vi "LinearSystemLoop_DiffDrv_Execute.vi"(5 "Linear System":T2, 6 "dT_Seconds":dbl=0.02 format="%#_13g", 7 "LinearSystemLoop_DiffDrv_Control_Params":T1={"Left Vel Model Std Dev m/s"=0.0, "Left Vel Meas Std Dev m/s"=0.0, "Left Vel Ctrl Tol m/s"=0.0, "Max Control Effort"=12.0, "Right Vel Ctrl Tol m/s"=0.0, "Right Vel Meas Std Dev m/s"=0.0, "Right Vel Model Std Dev m/s"=0.0}, 8 "Right Vel PV m/s":dbl, 9 "Left Vel PV m/s":dbl, 10 "Right Vel SP m/s":dbl, 11 "Left Vel SP m/s":dbl) -> (0 "Error":bool, 1 "Filtered Measurements":dbl[](array[numeric]), 2 "Right Motor Dmd":dbl, 3 "Left Motor Dmd":dbl, 4 "out Linear System Loop":T4)   [LabVIEW 2019, in "Trajectory_Library.lvlib"]
doc: "The linear system is define as:\n - states\n - left velocity (m/s)\n - right velocity (m/s)\n - inputs\n - left voltage (volts)\n - right voltage(volts)\n - outputs\n - left velocity (m/s)\n - right velocity (m/s)"
uses:
  Trajectory_Library.lvlib
  TypeDef/LINEAR_SYSTEM_LOOP.ctl
  TypeDef/LINEAR_QUADRATIC_REGULATOR.ctl
  <vilib>/Analysis/Matrix/Datatypes/RealMatrix.ctl
  TypeDef/LINEAR_PLANT_INV_FF.ctl
  TypeDef/KALMAN_FILTER.ctl
  TypeDef/LINEAR_SYSTEM.ctl
  TypeDef/LINEAR_SYSTEM_LOOP_DIFF_DRV_CTRL_PARAMS.CTL
  MatBuilder_Create.vi
  <vilib>/Analysis/Matrix/Numeric/Conversions/Matrix To Array - RM.vi
  <vilib>/Analysis/Matrix/NI_Matrix.lvlib
panel:
  # "<States,States>"
  # "<States,Inputs>"
  # "<Outputs,States>"
  # "<Outputs,Inputs>"
  # "<States,1>"
  # "<FUTURE --- CLAMP TYPE -- For now\nuse Normalize>"
  # "Steady State Gain  \n<States,Outputs>"
  # "State Estimate <Statess,1>"
  # "<States,States>"
  # "<States,Inputs>"
  # "<Outputs,States>"
  # "<Outputs,Inputs>"
  # "<States,1>"
  # "<Inputs,1>"
  # "<States,Inputs>"
  # "<States,States>"
  # "Ref State <States,1>"
  # "Comp and capped \noutput <Inputs,1>"
  # "Controller gain\n<Inputs,States>"
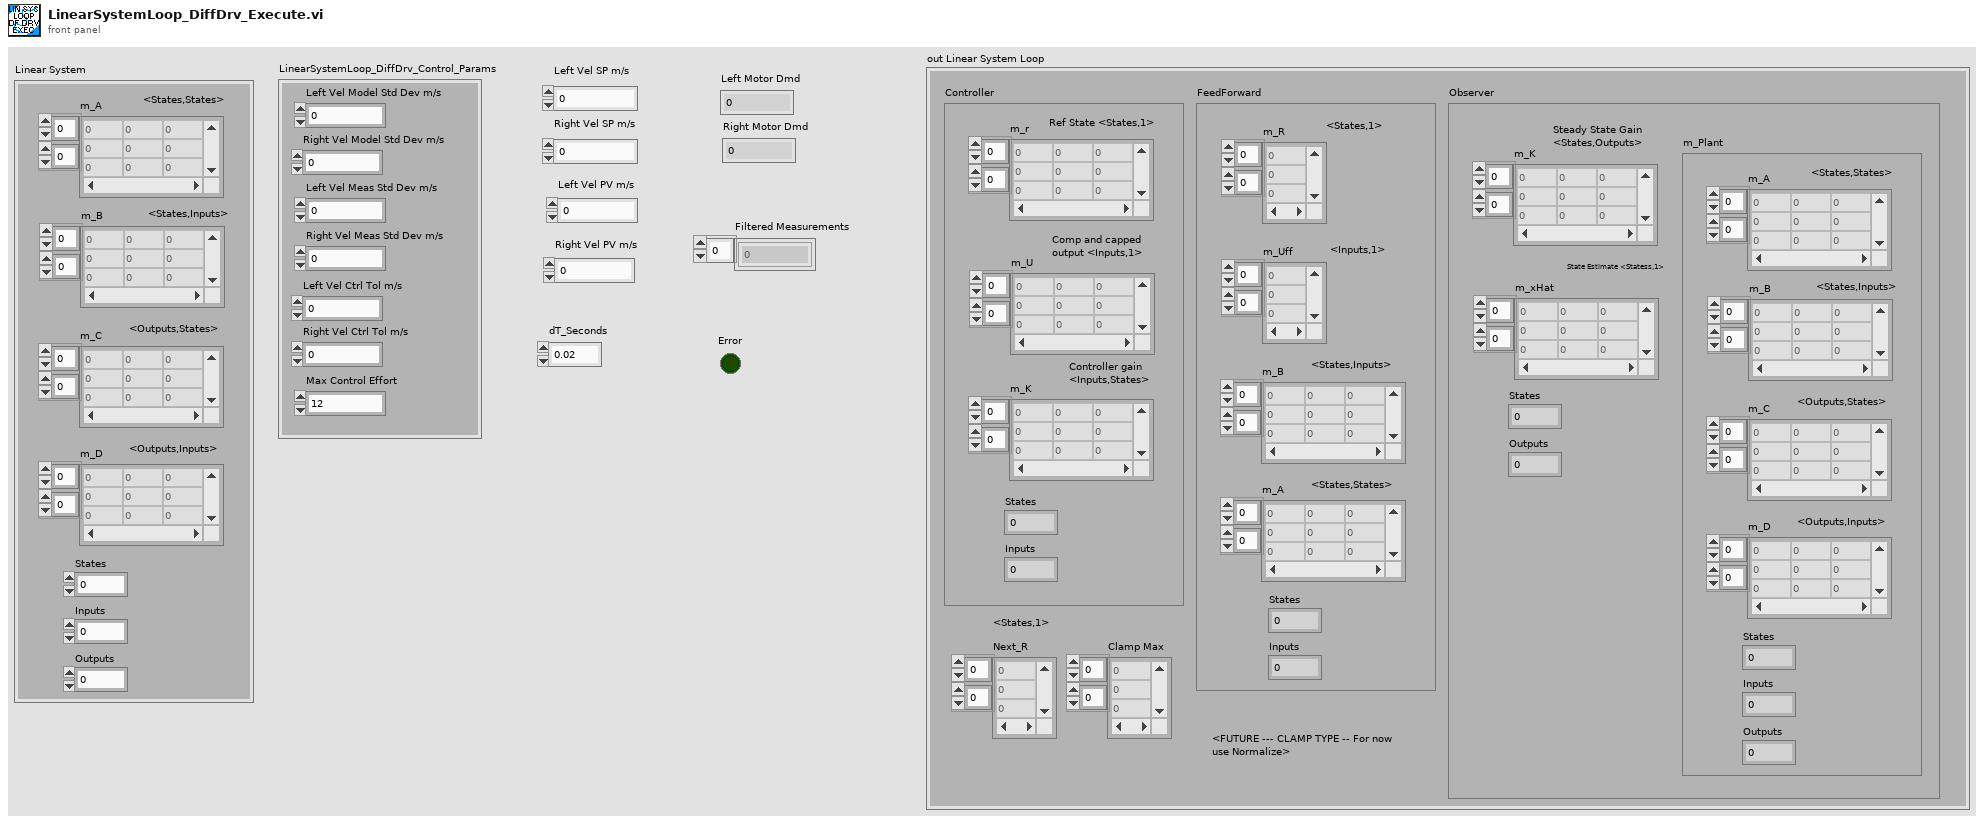
[diagram p1: front panel]
types:
  T1 = typedef "Trajectory_Library.lvlib/LINEAR_SYSTEM_LOOP_DIFF_DRV_CTRL_PARAMS.CTL" = cluster{"Left Vel Model Std Dev m/s":dbl, "Left Vel Meas Std Dev m/s":dbl, "Left Vel Ctrl Tol m/s":dbl, "Max Control Effort":dbl, "Right Vel Ctrl Tol m/s":dbl, "Right Vel Meas Std Dev m/s":dbl, "Right Vel Model Std Dev m/s":dbl}
  T2 = typedef "Trajectory_Library.lvlib/LINEAR_SYSTEM.ctl" = cluster{"m_A":T3, "m_B":T3, "m_C":T3, "m_D":T3, "States":i32, "Inputs":i32, "Outputs":i32}
  T3 = typedef "NI_Matrix.lvlib/RealMatrix.ctl" = dbl[][]
  T4 = typedef "Trajectory_Library.lvlib/LINEAR_SYSTEM_LOOP.ctl" = cluster{"Controller":T5, "FeedForward":T6, "Observer":T7, "Next_R":T3, "Clamp Max":T3}
  T5 = typedef "Trajectory_Library.lvlib/LINEAR_QUADRATIC_REGULATOR.ctl" = cluster{"m_r":T3, "m_U":T3, "m_K":T3, "States":i32, "Inputs":i32}
  T6 = typedef "Trajectory_Library.lvlib/LINEAR_PLANT_INV_FF.ctl" = cluster{"m_R":T3, "m_Uff":T3, "m_B":T3, "m_A":T3, "States":i32, "Inputs":i32}
  T7 = typedef "Trajectory_Library.lvlib/KALMAN_FILTER.ctl" = cluster{"m_K":T3, "m_xHat":T3, "States":i32, "Outputs":i32, "m_Plant":T2}
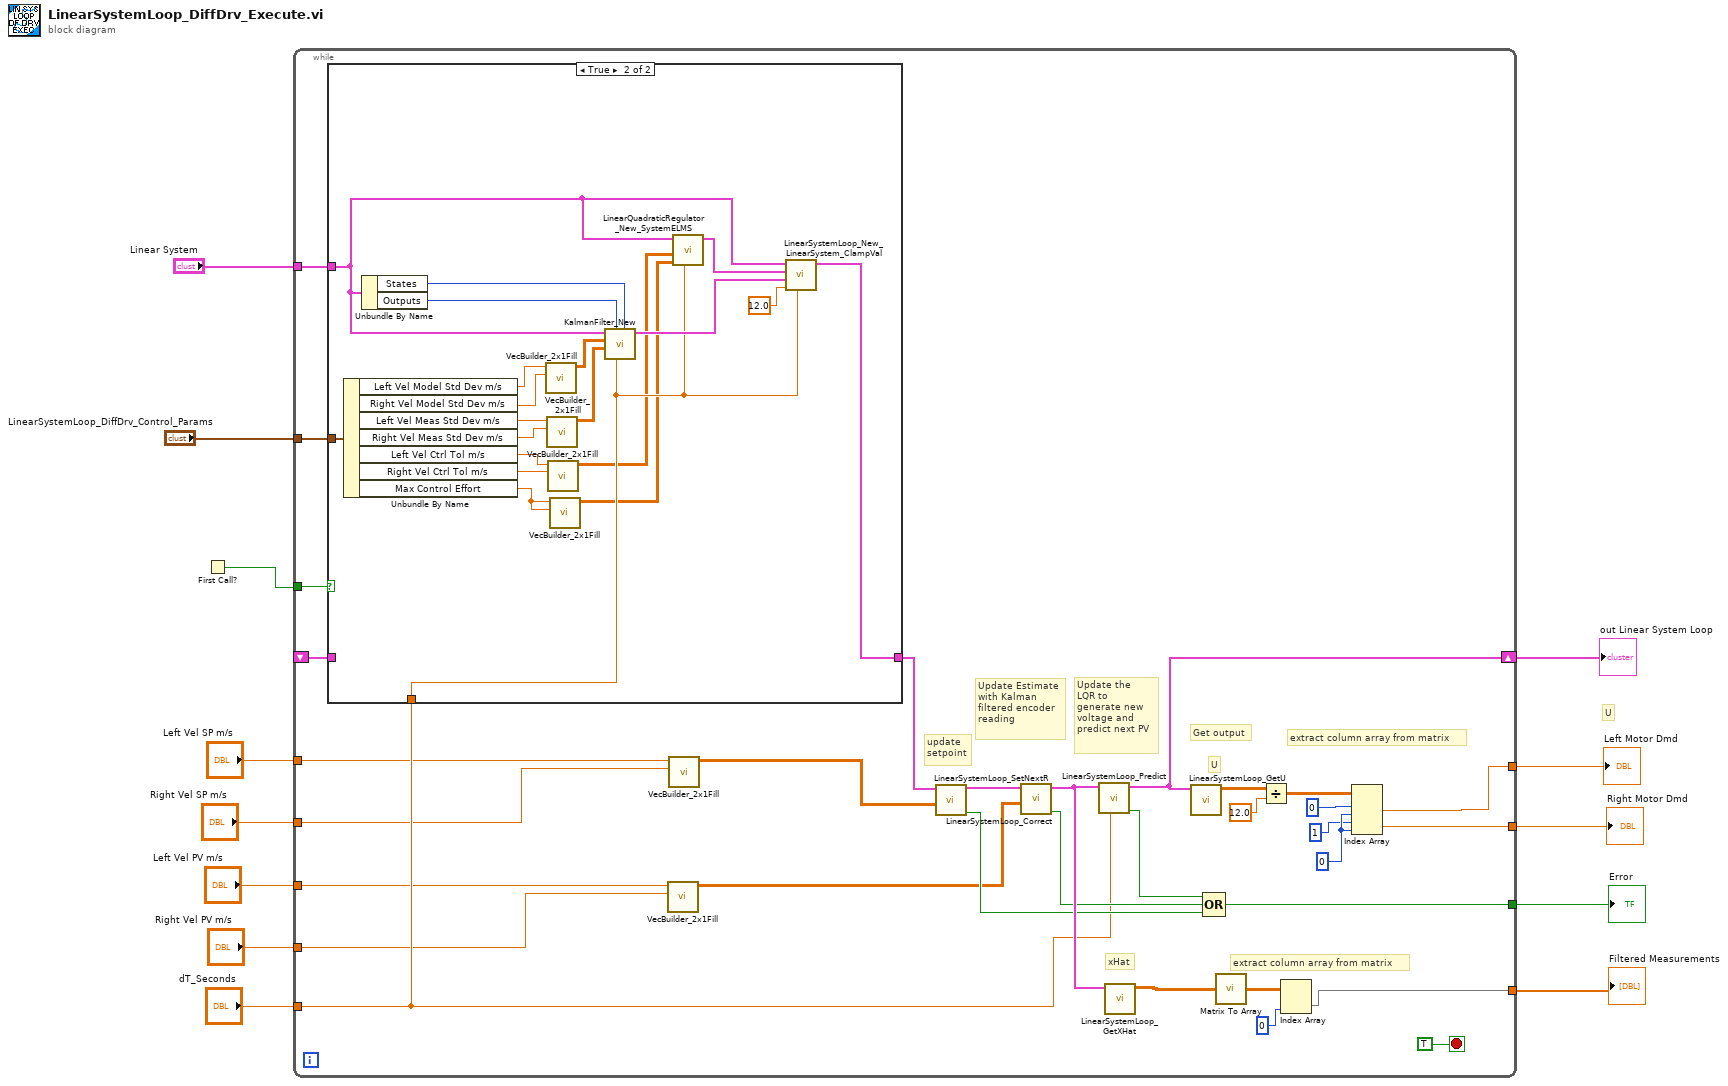
[diagram p0: block diagram]
diagram:
  # "U"
  n1 = First Call?() -> (First Call?: T/F=w9:bool)
  n2 = while {
    tunnel: [w40] -> w12
    tunnel: [w15] -> w7
    tunnel: "Left Vel SP m/s" -> [w24]
    tunnel: "Left Vel PV m/s" -> [w23]
    shift-right: [w44] -> w13
    shift-left: _ -> [w28]
    tunnel: w9 -> [w37]
    tunnel: [w34] -> w8
    tunnel: "dT_Seconds" -> [w29]
    tunnel: "Linear System" -> [w30]
    tunnel: "LinearSystemLoop_DiffDrv_Control_Params" -> [w26]
    tunnel: "Right Vel SP m/s" -> [w25]
    tunnel: "Right Vel PV m/s" -> [w22]
    tunnel: [w14] -> w1
    stop <- TRUE stop-if-true
    w18 = 0 ("index (col)")
    # "extract column array from matrix"
    # "extract column array from matrix"
    # "xHat"
    # "U"
    # "Get output"
    # "Update the \nLQR to \ngenerate new \nvoltage and \npredict next PV"
    # "update \nsetpoint"
    # "Update Estimate\nwith Kalman \nfiltered encoder \nreading"
    n3 = case shown="True" w37 {
      tunnel: [w46 w62] -> w27
      tunnel: w28 -> [w46 _]
      tunnel: w30 -> [_ w65]
      tunnel: w29 -> [_ w61]
      tunnel: w26 -> [_ w59]
      frame False {
      }
      frame True {
        n4 = Unbundle By Name(w59) -> ("Left Vel Model Std Dev m/s"=w57:dbl, "Right Vel Model Std Dev m/s"=w56:dbl, "Left Vel Meas Std Dev m/s"=w55:dbl, "Right Vel Meas Std Dev m/s"=w52:dbl, "Left Vel Ctrl Tol m/s"=w51:dbl, "Right Vel Ctrl Tol m/s"=w50:dbl, "Max Control Effort"=w49:dbl)
        n5 = Unbundle By Name(w65) -> ("States"=w58:i32, "Outputs"=w60:i32)
        n6 = call "VecBuilder_2x1Fill.vi"("R1"=w56, "R0"=w57) -> ("output matrix"=w54:T3)  [unwired: 9 in]
        n7 = call "VecBuilder_2x1Fill.vi"("R1"=w52, "R0"=w55) -> ("output matrix"=w53:T3)  [unwired: 9 in]
        n8 = call "VecBuilder_2x1Fill.vi"("R1"=w50, "R0"=w51) -> ("output matrix"=w48:T3)  [unwired: 9 in]
        n9 = call "VecBuilder_2x1Fill.vi"("R1"=w49, "R0"=w49) -> ("output matrix"=w47:T3)  [unwired: 9 in]
        n10 = call "KalmanFilter_New.vi"("States"=w58, "dt_Seconds"=w61, "Outputs"=w60, "MeasurementStdDevs"=w53, "StateStdDevs"=w54, "Plant"=w65) -> ("KalmanFilter"=w64:T7)  [unwired: 4 in, 1 out]
        n11 = call "LinearQuadraticRegulator_New_SystemELMS.vi"("dt_Seconds"=w61, "Relms"=w47, "Qelms"=w48, "LINEARSYSTEM"=w65) -> ("LinearQuadraticRegulator"=w66:T5)  [unwired: 6 in, 1 out]
        n12 = call "LinearSystemLoop_New_LinearSystem_ClampVal.vi"("dT_Seconds"=w61, "Max_Voltage"=12.0, "Observer"=w64, "Controller"=w66, "Plant"=w65) -> ("Linear System Loop"=w62:T4)  [unwired: 5 in, 1 out]
      }
    }
    n13 = call "VecBuilder_2x1Fill.vi"("R1"=w22, "R0"=w23) -> ("output matrix"=w20:T3)  [unwired: 9 in]
    n14 = call "VecBuilder_2x1Fill.vi"("R1"=w25, "R0"=w24) -> ("output matrix"=w21:T3)  [unwired: 9 in]
    n15 = call "LinearSystemLoop_SetNextR.vi"("R"=w21, "input inear System Loop"=w27) -> ("Size Coerced"=w31:bool, "out Linear System Loop"=w45:T4)  [unwired: 8 in]
    n16 = call "LinearSystemLoop_Correct.vi"("Y"=w20, "input inear System Loop"=w45) -> ("Error"=w41:bool, "out Linear System Loop"=w43:T4)  [unwired: 8 in]
    n17 = call "LinearSystemLoop_Predict.vi"("dT_Seconds"=w29, "input inear System Loop"=w43) -> ("Error"=w42:bool, "out Linear System Loop"=w44:T4)  [unwired: 8 in]
    n18 = call "LinearSystemLoop_GetXHat.vi"("input inear System Loop"=w43) -> ("XHat"=w32:T3)  [unwired: 10 in]
    n19 = call "LinearSystemLoop_GetU.vi"("input inear System Loop"=w44) -> ("U"=w39:T3)  [unwired: 10 in]
    n20 = Compound Arithmetic op=OR(w42, w41, w31) -> (w40:bool)
    n21 = call-poly <vilib>:"Matrix To Array.vi"("Real Matrix"=w32) -> ("Real 2D Array"=w36:dbl[][])
    n22 = Divide(x=w39, y=12.0) -> (x/y=w19:T3)
    n23 = Index Array(array=w36, index (col)=0 ("disabled index (col)")) -> (element=w34:dbl[])  [unwired: 1 in]
    n24 = Index Array(array=w19, index (row) #1=0 ("index (row)"), index (col) #1=w18, index (row) #2=1 ("index (row)"), index (col) #2=w18) -> (element #1=w15:dbl, element #2=w14:dbl)
  }
  "out Linear System Loop" <- w13
  "Error" <- w12
  "Filtered Measurements" <- w8
  "Left Motor Dmd" <- w7
  "Right Motor Dmd" <- w1
